vi "Setup Connection GUI.vi"(8 "error in (no error)":errorcluster, 9 "Mode Description Control":refnum<vi>, 10 "Connection Controls":refnum<vi>[](array[refnum]), 11 "Item Ref in":T6 format="%.0x") -> (0 "error out":errorcluster, 1 "ConSelection":T7, 2 "Connection Settings":T1, 3 "Item Ref out":T6 format="%.0x")   [LabVIEW 2017, in "Chassis TimeSync System Explorer.lvlib"]
uses:
  Chassis TimeSync System Explorer.lvlib
  <vilib>/NI Veristand/Custom Device API/Custom Device Item Ref.ctl
  Connection Selection.ctl
  Shared/Connection Settings.ctl
  Shared/Mode.ctl
  Shared/External Pin.ctl
  Shared/Routes.ctl
  Shared/Route.ctl
  sub_EnableDisable Controls.vi
  <vilib>/NI Veristand/Custom Device API/Custom Device API.lvlib
  Shared/Chassis TimeSync Shared.lvlib
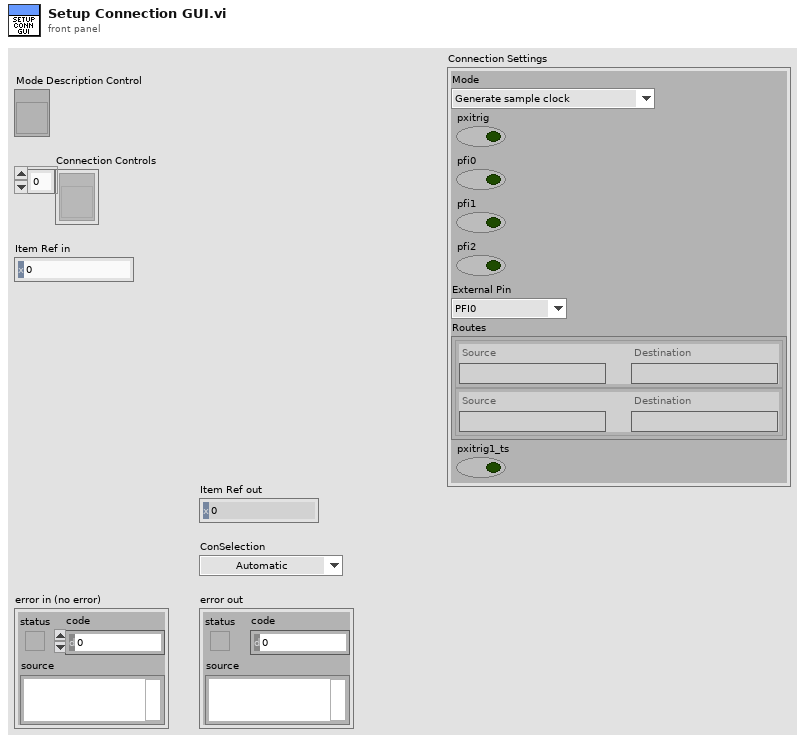
[diagram p1: front panel]
types:
  T1 = typedef "Chassis TimeSync Shared.lvlib/Connection Settings.ctl" = cluster{"Mode":T2, "pxitrig":bool, "pfi0":bool, "pfi1":bool, "pfi2":bool, "External Pin":T3, "Routes":T4, "pxitrig1_ts":bool}
  T2 = typedef "Chassis TimeSync Shared.lvlib/Mode.ctl" = enum16{"Generate sample clock", "Route sample clock out of chassis", "Route sample clock into chassis", "Custom routes"}
  T3 = typedef "Chassis TimeSync Shared.lvlib/External Pin.ctl" = enum16{"PFI0", "PFI1", "PFI2"}
  T4 = typedef "Chassis TimeSync Shared.lvlib/Routes.ctl" = T5[]
  T5 = typedef "Chassis TimeSync Shared.lvlib/Route.ctl" = cluster{"Source":string, "Destination":string}
  T6 = typedef "Custom Device API.lvlib/Custom Device Item Ref.ctl" = u64
  T7 = typedef "Chassis TimeSync System Explorer.lvlib/Connection Selection.ctl" = enum16{"Automatic", "Custom"}
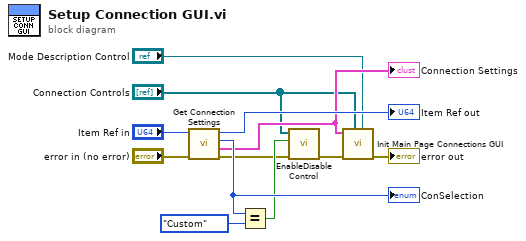
[diagram p0: block diagram]
diagram:
  n1 = call "Get Connection Settings.vi"("error in (no error)"="error in (no error)", "Item Ref in"="Item Ref in") -> ("error out"=w1:errorcluster, "Connection Settings"=w7:T1, "ConSelection"=w11:T7, "Item Ref out"=→"Item Ref out":T6)  [unwired: 6 in]
  "ConSelection" <- w11
  "Connection Settings" <- w7
  n2 = Equal?(x=w11, y=Connection_Selection."Custom") -> (x = y?=w10:bool)
  n3 = call-poly "EnableDisable Control.vi"("error in"=w1, "Enable"=w10, "Controls"="Connection Controls") -> ("error out"=w2:errorcluster)  [unwired: 8 in]
  n4 = call "Init Main Page Connections GUI.vi"("Mode Desciption"="Mode Description Control", "Controls"="Connection Controls", "error in (no error)"=w2, "AutoSelection"=w7) -> ("error out"=→"error out":errorcluster)  [unwired: 7 in]
